vi "Magnetic Field Lakeshore Continuous.vi"(8 "error in (no error)":errorcluster, 10 "Lakeshore Gaussmeter.lvclass":refnum<class "Lakeshore Gaussmeter.lvclass">, 11 "Magnetic Field Lakeshore Continuous.lvclass in":refnum<class "Magnetic Field Lakeshore Continuous.lvclass">) -> (0 "error out":errorcluster, 3 "Magnetic Field Lakeshore Continuous.lvclass out":refnum<class "Magnetic Field Lakeshore Continuous.lvclass">)   [LabVIEW 2017, in "Magnetic Field Lakeshore Continuous.lvclass"]
uses:
  Magnetic Field Lakeshore Continuous.lvclass
  C:/LabVIEW-programs/Scanners/Scanner/Scanner.lvclass
  Instruments/Lakeshore Gaussmeter/Lakeshore Gaussmeter.lvclass
  C:/LabVIEW-programs/Instruments/Utility Classes/Scannable/Scannable.lvclass
  Magnetic Field Lakeshore Continuous.lvclass/Magnetic Field Lakeshore Continuous.ctl
  Scanner/Scanner.lvclass
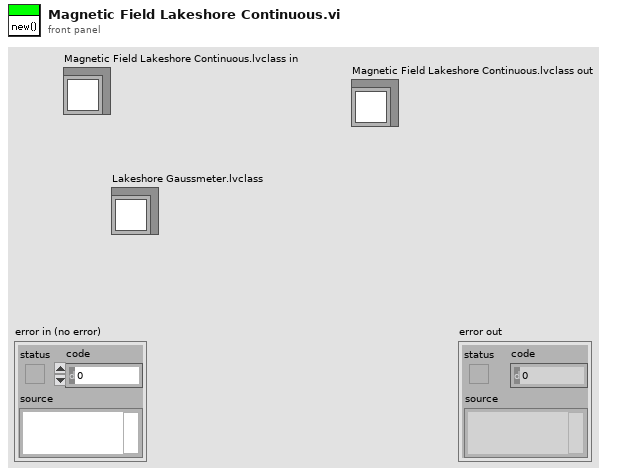
[diagram p1: front panel]
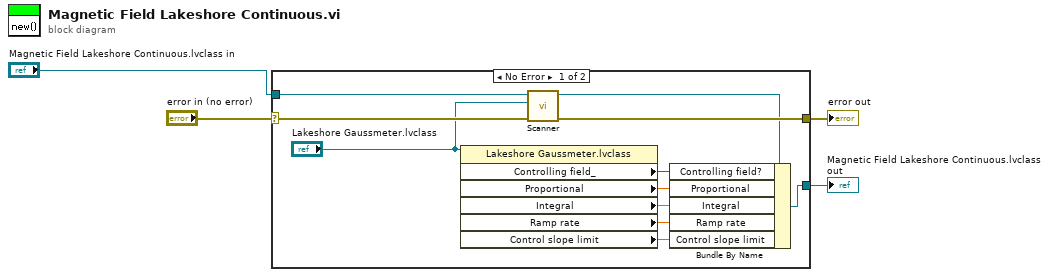
[diagram p0: block diagram]
diagram:
  n1 = case shown="No Error" "error in (no error)" {
    selector: "error in (no error)" -> [w15 w17]
    tunnel: [w14 w17] -> w3
    tunnel: "Magnetic Field Lakeshore Continuous.lvclass in" -> [w13 w16]
    tunnel: [w10 w16] -> w1
    frame No Error {
      n2 = property class="Lakeshore Gaussmeter.lvclass"(reference="Lakeshore Gaussmeter.lvclass") -> ("Controlling field_"=w9:bool, "Proportional"=w8:dbl, "Integral"=w7:dbl[unit], "Ramp rate"=w6:dbl[unit], "Control slope limit"=w5:dbl[unit])  [unwired: 1 in, 2 out]
      n3 = call "Scanner.vi"("error in (no error)"=w15, "Scannable"="Lakeshore Gaussmeter.lvclass", "Scanner.lvclass in"=w13) -> ("error out"=w14:errorcluster, "Scanner.lvclass out"=w11:refnum<class "Magnetic Field Lakeshore Continuous.lvclass">)  [unwired: 1 in, 6 out]
      n4 = Bundle By Name(cluster=w11, "Controlling field?"=w9, "Proportional"=w8, "Integral"=w7, "Ramp rate"=w6, "Control slope limit"=w5) -> (w10:refnum<class "Magnetic Field Lakeshore Continuous.lvclass">)
    }
    frame Error {
    }
  }
  "error out" <- w3
  "Magnetic Field Lakeshore Continuous.lvclass out" <- w1
